vi "niRFUtil RFHS Util Process CPU Context.vi"(0 "CPU Context":T2 format="%.0x", 5 "Points":i32, 7 "Threshold":i32, 9 "Multiple":i32) -> (4 "Exec Config":T1 {"CPU Context" format="%.0x"}, 6 "First Points":i32[](array[numeric]))   [LabVIEW 2015, in "niRFUtil.lvlib"]
uses:
  niRFUtil.lvlib
  niRFUtil RFHS Util CPU Context.ctl
  Channelizer/Includes/niRFUtil RFHS Channelizer CPUInfo.ctl
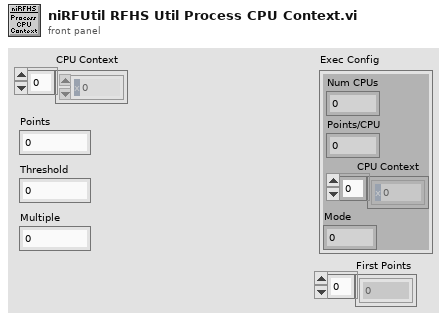
[diagram p1: front panel]
types:
  T1 = typedef "niRFUtil.lvlib/niRFUtil RFHS Channelizer CPUInfo.ctl" = cluster{"Num CPUs":u32, "Points/CPU":u32, "CPU Context":T2, "Mode":i32}
  T2 = typedef "niRFUtil.lvlib/niRFUtil RFHS Util CPU Context.ctl" = u64[]
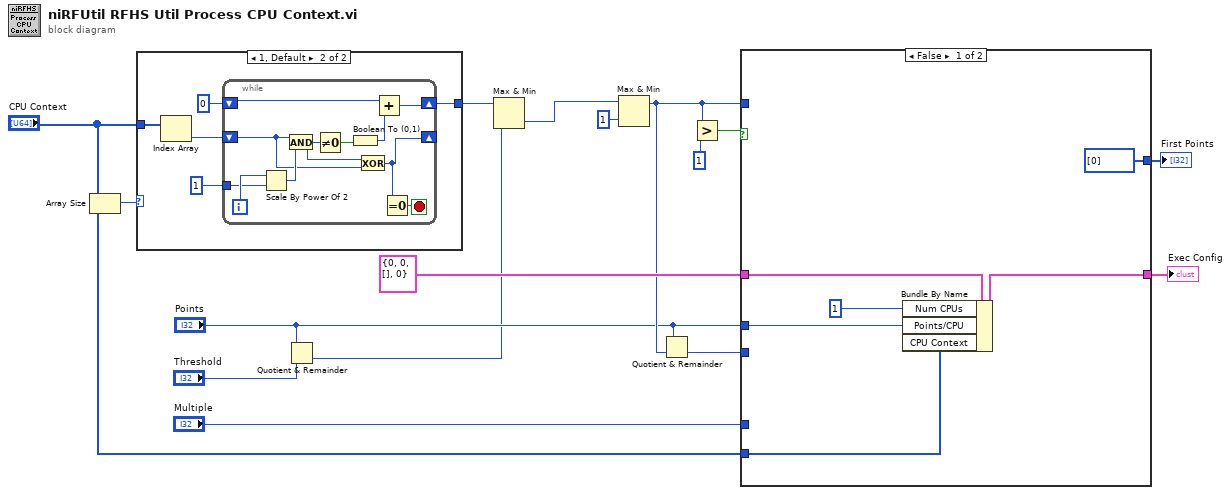
[diagram p0: block diagram]
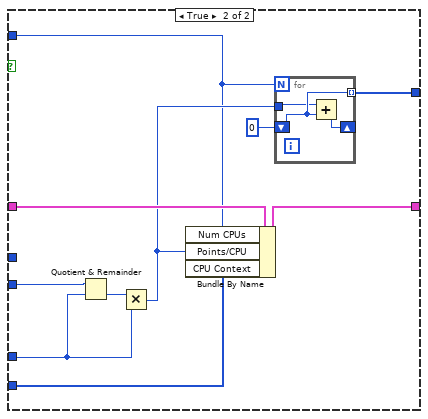
[diagram p2: hidden frame]
diagram:
  n1 = Array Size(array="CPU Context") -> (size(s)=w16:i32)
  n2 = case shown="1, Default" w16 {
    tunnel: "CPU Context" -> [_ w21]
    tunnel: [_ w17] -> w7
    frame 0 {
    }
    frame 1, Default {
      n3 = Index Array(array=w21) -> (element=w20:u64)  [unwired: 1 in]
      n4 = while {
        tunnel: u64 1 -> [w31]
        shift-right: [w28] -> w17
        shift-left: 0 -> [w29]
        shift-right: [w23] -> _
        shift-left: w20 -> [w24]
        i -> [w32]
        stop <- w22 stop-if-true
        n5 = Scale By Power Of 2(n=w32, x=w31) -> (x*2^n=w30:u64)
        n6 = And(x=w24, y=w30) -> (x .and. y?=w25:u64)
        n7 = Not Equal To 0?(x=w25) -> (x != 0?=w26:bool)
        n8 = Boolean To (0,1)(Boolean=w26) -> (0, 1=w27:i16)
        n9 = Exclusive Or(1:w24, 2:w25) -> (0:w23:u64)
        n10 = Add(x=w29, y=w27) -> (x+y=w28:i32)
        n11 = Equal To 0?(x=w23) -> (x = 0?=w22:bool)
      }
    }
  }
  n12 = Quotient & Remainder(x="Points", y="Threshold") -> (floor(x/y)=w6:i32)  [unwired: 1 out]
  n13 = Max & Min(x=w7, y=w6) -> (min(x,y)=w5:i32)  [unwired: 1 out]
  n14 = Max & Min(x=w5, y=1) -> (max(x,y)=w11:i32)  [unwired: 1 out]
  n15 = Quotient & Remainder(x="Points", y=w11) -> (floor(x/y)=w10:i32)  [unwired: 1 out]
  n16 = Greater?(x=w11, y=1) -> (0:w3:bool)
  n17 = case shown="False" w3 {
    tunnel: T1 {"Num CPUs"=0, "Points/CPU"=0, "CPU Context"=[], "Mode"=0} ("Exec Config") -> [w38 w45]
    tunnel: "Points" -> [w36 _]
    tunnel: [w35 w44] -> w13
    tunnel: w11 -> [_ w40]
    tunnel: w10 -> [_ w48]
    tunnel: "Multiple" -> [_ w46]
    tunnel: "CPU Context" -> [w33 w43]
    tunnel: [i32[] [0] w39] -> w1
    frame False {
      n18 = Bundle By Name(cluster=w38, "Num CPUs"=u32 1, "Points/CPU"=w36, "CPU Context"=w33) -> (w35:T1)
    }
    frame True {
      n19 = Quotient & Remainder(x=w48, y=w46) -> (floor(x/y)=w47:i32)  [unwired: 1 out]
      n20 = Multiply(x=w47, y=w46) -> (x*y=w42:i32)
      n21 = Bundle By Name(cluster=w45, "Num CPUs"=w40, "Points/CPU"=w42, "CPU Context"=w43) -> (w44:T1)
      n22 = for {
        N: w40 -> [_]
        tunnel: w42 -> [w50]
        shift-right: [w49] -> _
        shift-left: 0 -> [w51]
        tunnel: [w51] -> w39 mode=indexing
        n23 = Add(x=w50, y=w51) -> (x+y=w49:i32)
      }
    }
  }
  "Exec Config" <- w13
  "First Points" <- w1
